vi "wcs_rotate.vi"(8 "latitude":dbl format="%_8g", 9 "longitude":dbl, 11 "Astrometry":T1) -> (0 "theta":dbl, 1 "phi":dbl)   [LabVIEW 2019]
panel:
  out "cp":dbl format="%_6g"
  out "sp":dbl format="%_6g"
  out "cd":dbl
  out "sd":dbl
  out "ca":dbl
  out "sa":dbl
  out "delta_p":dbl
  out "alpha_p":dbl
  out "b2":dbl
  out "b0":dbl
  out "b1":dbl
  out "theta1":dbl format="%#.8g"
  out "phi1":dbl
  out "n":dbl
  out "m":dbl
  out "l":dbl
  out "rr":dbl[][](array[numeric])
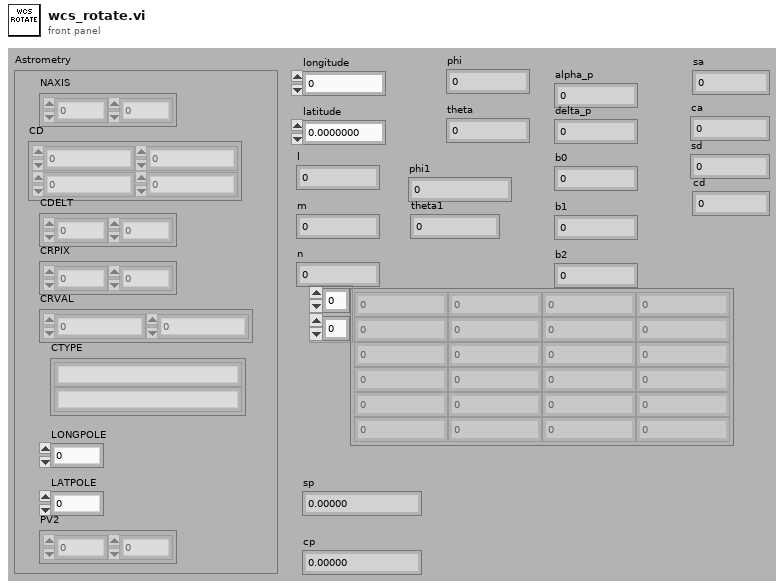
[diagram p1: front panel]
types:
  T1 = cluster{"NAXIS":dbl[], "CD":dbl[][], "CDELT":dbl[], "CRPIX":dbl[], "CTYPE":string[], "CRVAL":dbl[], "LONGPOLE":dbl, "LATPOLE":dbl, "PV2":dbl[]}
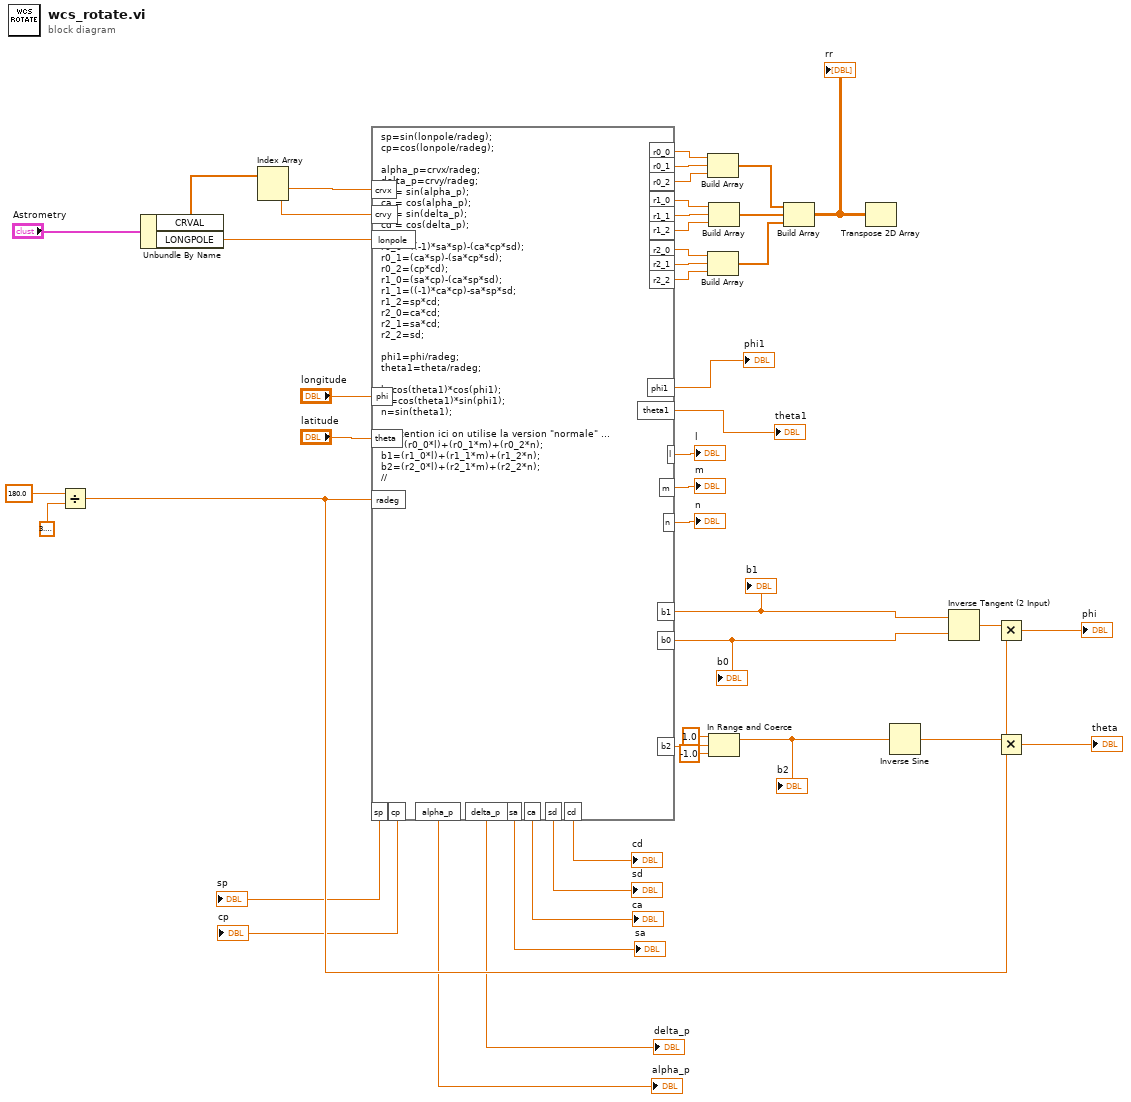
[diagram p0: block diagram]
diagram:
  n1 = Divide(x=180.0, y=3.141592653589793) -> (x/y=w17:dbl)
  n2 = Unbundle By Name("Astrometry") -> ("CRVAL"=w45:dbl[], "LONGPOLE"=w1:dbl)
  n3 = Index Array(array=w45) -> (element #1=w44:dbl, element #2=w43:dbl)  [unwired: 2 in]
  n4 = formula code="sp=sin(lonpole/radeg);\ncp=cos(lonpole/radeg);\n\nalpha_p=crvx/radeg;\ndelta_p=crvy/radeg;\nsa = sin(alpha_p);\nca = cos(alpha_p);\nsd = sin(delta_p);\ncd = cos(delta_p);\n\nr0_0=((-1)*sa*sp)-(ca*cp*sd);\nr0_1=(ca*sp)-(sa*cp*sd);\nr0_2=(cp*cd);\nr1_0=(sa*cp)-(ca*sp*sd);\nr1_1=((-1)*ca*cp)-sa*sp*sd;\nr1_2=sp*cd;\nr2_0=ca*cd;\nr2_1=sa*cd;\nr2_2=sd;\n\nphi1=phi/radeg;\ntheta1=theta/radeg;\n\nl=cos(theta1)*cos(phi1);\nm=cos(theta1)*sin(phi1);\nn=sin(theta1);\n\n// Attention ici on utilise la version \"normale\" ...\nb0 =(r0_0*l)+(r0_1*m)+(r0_2*n);\nb1=(r1_0*l)+(r1_1*m)+(r1_2*n);\nb2=(r2_0*l)+(r2_1*m)+(r2_2*n);\n//"("lonpole"=w1, "crvx"=w44, "crvy"=w43, "radeg"=w17, "phi"="longitude", "theta"="latitude") -> ("sp"=→"sp":dbl, "cp"=→"cp":dbl, "sa"=→"sa":dbl, "ca"=→"ca":dbl, "sd"=→"sd":dbl, "cd"=→"cd":dbl, "r0_0"=w42:dbl, "r0_1"=w41:dbl, "r0_2"=w40:dbl, "r1_0"=w39:dbl, "r1_1"=w38:dbl, "r1_2"=w37:dbl, "r2_0"=w36:dbl, "r2_1"=w35:dbl, "r2_2"=w34:dbl, "alpha_p"=→"alpha_p":dbl, "delta_p"=→"delta_p":dbl, "phi1"=→"phi1":dbl, "theta1"=→"theta1":dbl, "l"=→"l":dbl, "m"=→"m":dbl, "n"=→"n":dbl, "b0"=w19:dbl, "b1"=w20:dbl, "b2"=w13:dbl)
  "b1" <- w20
  "b0" <- w19
  n5 = Build Array(w42, w41, w40) -> (w33:dbl[])
  n6 = Build Array(w36, w35, w34) -> (w31:dbl[])
  n7 = Build Array(w39, w38, w37) -> (w32:dbl[])
  n8 = In Range and Coerce(upper limit=1.0, x=w13, lower limit=-1.0) -> (coerced(x)=w10:dbl)  [unwired: 1 out]
  "b2" <- w10
  n9 = Build Array(w33, w32, w31) -> (w28:dbl[][])
  "rr" <- w28
  n10 = Transpose 2D Array(2D array=w28) -> ()  [unwired: 1 out]
  n11 = Inverse Sine(1:w10) -> (0:w22:dbl)
  n12 = Inverse Tangent (2 Input)(1:w19, 2:w20) -> (0:w18:dbl)
  n13 = Multiply(x=w18, y=w17) -> (x*y=→"phi":dbl)
  n14 = Multiply(x=w22, y=w17) -> (x*y=→"theta":dbl)
